vi "AxisEnumToAxisInfo.vi"(11 "Motor Axis":T2) -> (0 "Axis ID":string[](array[string]), 1 "System #":i32, 2 "Valid axis?":bool, 3 "Axis info":T1={"System #"=0, "Axis ID"="", "Multiplier"=1.0}, 4 "Multiplier":dbl)   [LabVIEW 2011]
uses:
  Main/Motors/MotorAxisEnum.ctl
  PI_Axis.ctl
  PIAxisInfoGlobal.vi
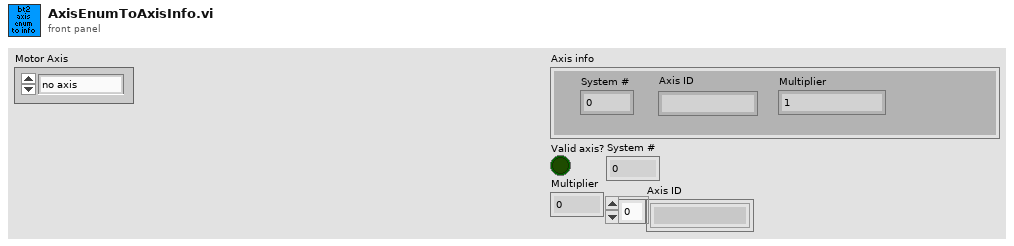
[diagram p1: front panel]
types:
  T1 = typedef "PI_Axis.ctl" = cluster{"System #":i32, "Axis ID":string, "Multiplier":dbl}
  T2 = typedef "MotorAxisEnum.ctl" = enum16{"no axis", "magrot", "magpos", "px", "py", "pz", "camx", "camy"}
  T3 = typedef "PI_Axis_list.ctl" = cluster{"Piezo X":T1, "Piezo Y":T1, "Piezo Z":T1, "Magnet Z":T1, "Magnet Rotation":T1, "Objective X":T1, "Objective Y":T1}
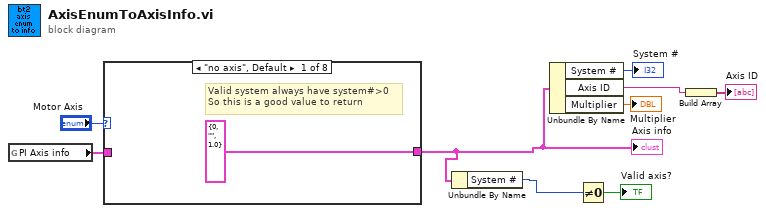
[diagram p0: block diagram]
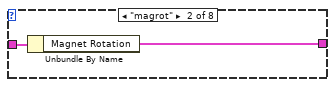
[diagram p2: hidden frame]
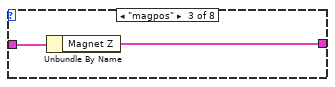
[diagram p3: hidden frame]
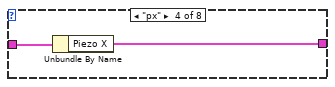
[diagram p4: hidden frame]
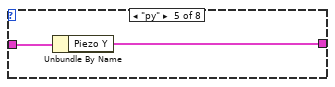
[diagram p5: hidden frame]
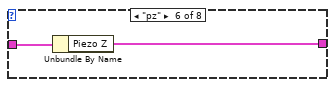
[diagram p6: hidden frame]
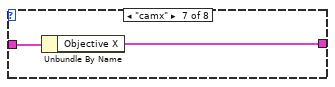
[diagram p7: hidden frame]
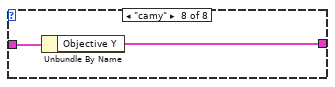
[diagram p8: hidden frame]
diagram:
  n1 = global read "PIAxisInfoGlobal.vi" "PI Axis info"() -> (w8:T3)
  n2 = case shown="\"no axis\", Default" "Motor Axis" {
    tunnel: w8 -> [_ w12 w14 w16 w18 w20 w22 w24]
    tunnel: [T1 {"System #"=0, "Axis ID"="", "Multiplier"=1.0} ("Magnet Rotation") w11 w13 w15 w17 w19 w21 w23] -> w5
    frame "no axis", Default {
      # "Valid system always have system#>0\nSo this is a good value to return"
    }
    frame "magrot" {
      n3 = Unbundle By Name(w12) -> ("Magnet Rotation"=w11:T1)
    }
    frame "magpos" {
      n4 = Unbundle By Name(w14) -> ("Magnet Z"=w13:T1)
    }
    frame "px" {
      n5 = Unbundle By Name(w16) -> ("Piezo X"=w15:T1)
    }
    frame "py" {
      n6 = Unbundle By Name(w18) -> ("Piezo Y"=w17:T1)
    }
    frame "pz" {
      n7 = Unbundle By Name(w20) -> ("Piezo Z"=w19:T1)
    }
    frame "camx" {
      n8 = Unbundle By Name(w22) -> ("Objective X"=w21:T1)
    }
    frame "camy" {
      n9 = Unbundle By Name(w24) -> ("Objective Y"=w23:T1)
    }
  }
  "Axis info" <- w5
  n10 = Unbundle By Name(w5) -> ("System #"=w7:i32)
  n11 = Unbundle By Name(w5) -> ("System #"=→"System #":i32, "Axis ID"=w3:string, "Multiplier"=→"Multiplier":dbl)
  n12 = Not Equal To 0?(x=w7) -> (x != 0?=→"Valid axis?":bool)
  n13 = Build Array(w3) -> (→"Axis ID":string[])
